vi "map_pixels.vi"(7 "Image size":T1=128 items=["128x128 px"=128, "256x256 px"=256, "512x512 px"=512], 8 "error in":errorcluster, 10 "Stream in":dbl[](array[numeric]), 11 "Lookup arrays":T2) -> (0 "error out":errorcluster, 3 "Image out":dbl[][](array[numeric]))   [LabVIEW 2011, in "Fiberscope_library.lvlib"]
uses:
  Fiberscope_library.lvlib
  typedefs/lookup_arrays_ref_cluster.ctl
  typedefs/image_size_I32.ctl
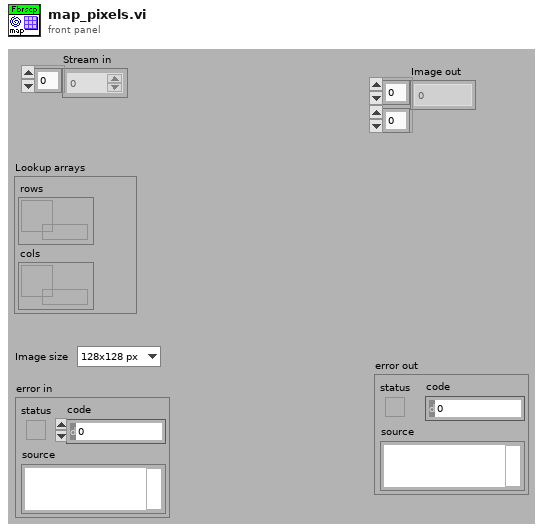
[diagram p1: front panel]
types:
  T1 = typedef "Fiberscope_library.lvlib/image_size_I32.ctl" = i32
  T2 = typedef "Fiberscope_library.lvlib/lookup_arrays_ref_cluster.ctl" = cluster{"rows":refnum<data-value>, "cols":refnum<data-value>}
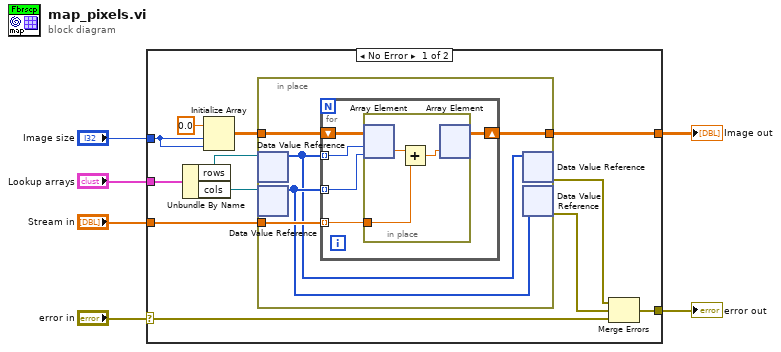
[diagram p0: block diagram]
diagram:
  n1 = case shown="No Error" "error in" {
    selector: "error in" -> [w15 w32]
    tunnel: [w14 w32] -> w5
    tunnel: "Stream in" -> [w17 _]
    tunnel: "Image size" -> [w18 _]
    tunnel: "Lookup arrays" -> [w16 _]
    tunnel: [w13 _] -> w2
    frame No Error {
      n2 = Unbundle By Name(w16) -> ("rows"=w10:refnum<data-value>, "cols"=w9:refnum<data-value>)
      n3 = Initialize Array(0.0 ("element"), w18, w18) -> (w11:dbl[][])
      n4 = in-place {
        in-place-border: w11 -> [w23]
        in-place-border: w17 -> [w22]
        in-place-border: [w19] -> w13
        n5 = in-place-dvr #1(w10) -> (w20:i32[])  [unwired: 1 out]
        n6 = in-place-dvr #2(w9) -> (w21:i32[])  [unwired: 1 out]
        n7 = for {
          shift-right: [w24] -> w19
          shift-left: w23 -> [w28]
          tunnel: w22 -> [w25] mode=indexing
          tunnel: w20 -> [w27] mode=indexing
          tunnel: w21 -> [w26] mode=indexing
          n8 = in-place {
            in-place-border: w25 -> [w30]
            n9 = in-place-array #3(w28, w27, w26) -> (w31:dbl)
            n10 = Add(x=w31, y=w30) -> (x+y=w29:dbl)
            n11 = in-place-array #3(w29) -> (w24:dbl[][])  [unwired: 2 out]
          }
        }
        n12 = in-place-dvr #1(w20) -> (w7:errorcluster)  [unwired: 1 out]
        n13 = in-place-dvr #2(w21) -> (w8:errorcluster)  [unwired: 1 out]
      }
      n14 = Merge Errors(w7, w8, w15) -> (w14:errorcluster)
    }
    frame Error {
    }
  }
  "error out" <- w5
  "Image out" <- w2
